vi "Final_Write_Key.vi"(7 "AllObjs[]":refnum<vi>[](array[refnum]), 8 "error in (no error)":errorcluster, 9 "Label.Text":string, 10 "String":string, 11 "Refnum in":T1) -> (0 "error out":errorcluster, 3 "Refnum out":T1)   [LabVIEW 2014]
uses:
  <vilib>/Utility/config.llb/Config Data RefNum.ctl
  <vilib>/Utility/config.llb/Write Key (Double).vi
  <vilib>/Utility/config.llb/Write Key (String).vi
  <vilib>/Utility/config.llb/Write Key (Path).vi
  <vilib>/Utility/config.llb/Write Key (I32).vi
  <vilib>/Utility/config.llb/Write Key (U32).vi
  <vilib>/Utility/config.llb/Write Key (Boolean).vi
  <vilib>/Utility/config.llb/NI_LVConfig.lvlib
  <vilib>/Utility/VariantDataType/VariantType.lvlib
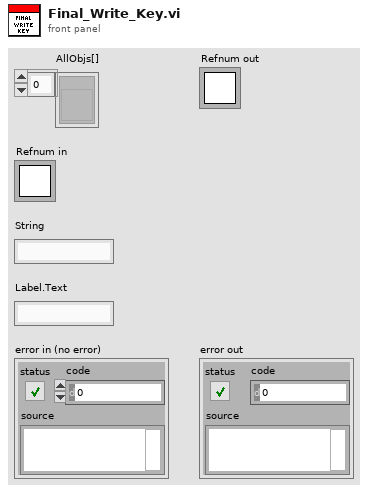
[diagram p1: front panel]
types:
  T1 = typedef "NI_LVConfig.lvlib/Config Data RefNum.ctl" = refnum<k1>
  T2 = typedef "VariantType.lvlib/Type.ctl" = enum8{"Invalid Type", "Void", "I8", "I16", "I32", "I64", "U8", "U16", "U32", "U64", "Single Float", "Double Float", "Extended Float", "Single Complex", "Double Complex", "Extended Complex", "Enum U8", "Enum U16", "Enum U32", "Enum U64", "Single Float With Unit", "Double Float With Unit", "Extended Float With Unit", "Single Complex with Unit", "Double Complex with Unit", "Extended Complex with Unit", "Boolean", "String", "Path", "Picture", "Tag", "Array", "Cluster", "Variant", "LV Variant", "Waveform", "Timestamp", "Digital Waveform", "Digital Data", "ExpressData", "Refnum", "External Data", "VI", "Poly VI", "LabVIEW Class Instance", "Fixed Point"}
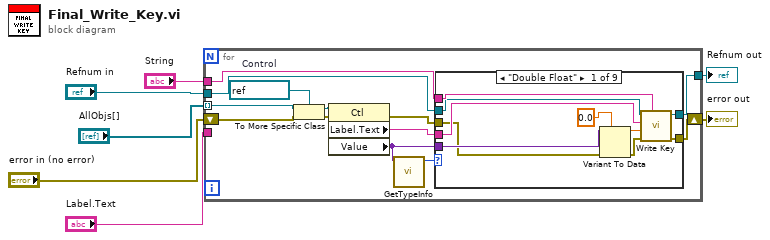
[diagram p0: block diagram]
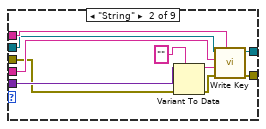
[diagram p2: hidden frame]
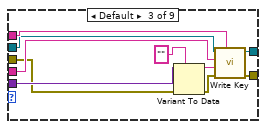
[diagram p3: hidden frame]
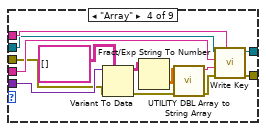
[diagram p4: hidden frame]
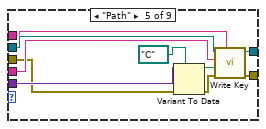
[diagram p5: hidden frame]
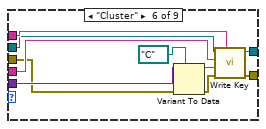
[diagram p6: hidden frame]
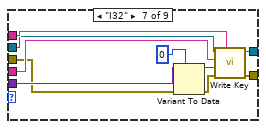
[diagram p7: hidden frame]
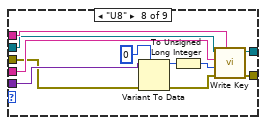
[diagram p8: hidden frame]
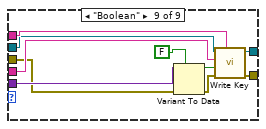
[diagram p9: hidden frame]
diagram:
  n1 = for {
    tunnel: "String" -> [w20]
    tunnel: [w19] -> w1
    tunnel: "Refnum in" -> [w15]
    tunnel: "AllObjs[]" -> [w11] mode=indexing
    tunnel: "Label.Text" -> [_]
    shift-right: [w18] -> w2
    shift-left: "error in (no error)" -> [w10]
    w17 = refnum<vi> refnum  # Control
    n2 = To More Specific Class(target class=w17, reference=w11, error in=w10) -> (specific class reference=w16:refnum<vi>, error out=w9:errorcluster)
    n3 = property class="Ctl"(reference=w16, error in=w9) -> (error out=w8:errorcluster, "Label.Text"=w12:string, "Value"=w13:variant)  [unwired: 1 out]
    n4 = call <vilib>:"GetTypeInfo.vi"("Variant"=w13) -> ("Type Enum"=w14:T2)  [unwired: 6 in, 4 out]
    n5 = case shown="\"Double Float\"" w14 {
      tunnel: w20 -> [w30 w40 w50 w63 w67 w83 w93 w104 w114]
      tunnel: w12 -> [w29 w39 w43 w62 w66 w82 w92 w103 w113]
      tunnel: w13 -> [w28 w38 w49 w61 w73 w81 w91 w102 w112]
      tunnel: w15 -> [w23 w33 w44 w56 w68 w76 w85 w96 w107]
      tunnel: [w27 w37 w48 w60 w72 w80 w90 w101 w111] -> w18
      tunnel: [w26 w36 w47 w59 w71 w79 w89 w100 w110] -> w19
      tunnel: w8 -> [w22 w32 w42 w53 w65 w75 w84 w95 w106]
      frame "Double Float" {
        n6 = Variant To Data(error in=w22, type=0.0, Variant=w28) -> (data=w24:dbl, error out=w21:errorcluster)
        n7 = call-poly <vilib>:"Write Key.vi"("section"=w30, "error in (no error)"=w21, "value"=w24, "key"=w29, "refnum"=w23) -> ("error out"=w27:errorcluster, "refnum out"=w26:T1)  [unwired: 4 in, 1 out]
      }
      frame "String" {
        n8 = Variant To Data(error in=w32, type="" ("Label.Text"), Variant=w38) -> (data=w34:string, error out=w31:errorcluster)
        n9 = call-poly <vilib>:"Write Key.vi"("section"=w40, "error in (no error)"=w31, "value"=w34, "key"=w39, "refnum"=w33) -> ("error out"=w37:errorcluster, "refnum out"=w36:T1)  [unwired: 4 in, 1 out]
      }
      frame Default {
        n10 = Variant To Data(error in=w42, type="" ("Label.Text"), Variant=w49) -> (data=w45:string, error out=w41:errorcluster)
        n11 = call-poly <vilib>:"Write Key.vi"("section"=w50, "error in (no error)"=w41, "value"=w45, "key"=w43, "refnum"=w44) -> ("error out"=w48:errorcluster, "refnum out"=w47:T1)  [unwired: 4 in, 1 out]
      }
      frame "Array" {
        n12 = Variant To Data(error in=w53, type=string[][] [], Variant=w61) -> (data=w57:string[][], error out=w52:errorcluster)
        n13 = Fract/Exp String To Number(string=w57) -> (number=w55:dbl[][])  [unwired: 3 in, 1 out]
        n14 = call "UTILITY DBL Array to String Array.vi"("Error in (no error)"=w52, "Array in"=w55) -> ("Error out"=w51:errorcluster, "String array out"=w54:string)  [unwired: 8 in]
        n15 = call-poly <vilib>:"Write Key.vi"("section"=w63, "error in (no error)"=w51, "value"=w54, "key"=w62, "refnum"=w56) -> ("error out"=w60:errorcluster, "refnum out"=w59:T1)  [unwired: 4 in, 1 out]
      }
      frame "Path" {
        n16 = Variant To Data(error in=w65, type=path "C:/" ("configuration file path 2"), Variant=w73) -> (data=w69:path, error out=w64:errorcluster)
        n17 = call-poly <vilib>:"Write Key.vi"("section"=w67, "error in (no error)"=w64, "value"=w69, "key"=w66, "refnum"=w68) -> ("error out"=w72:errorcluster, "refnum out"=w71:T1)  [unwired: 4 in, 1 out]
      }
      frame "Cluster" {
        n18 = Variant To Data(error in=w75, type=path "C:/" ("configuration file path 2"), Variant=w81) -> (data=w77:path, error out=w74:errorcluster)
        n19 = call-poly <vilib>:"Write Key.vi"("section"=w83, "error in (no error)"=w74, "value"=w77, "key"=w82, "refnum"=w76) -> ("error out"=w80:errorcluster, "refnum out"=w79:T1)  [unwired: 4 in, 1 out]
      }
      frame "I32" {
        n20 = Variant To Data(error in=w84, type=0, Variant=w91) -> (data=w86:i32, error out=w87:errorcluster)
        n21 = call-poly <vilib>:"Write Key.vi"("section"=w93, "error in (no error)"=w87, "value"=w86, "key"=w92, "refnum"=w85) -> ("error out"=w90:errorcluster, "refnum out"=w89:T1)  [unwired: 4 in, 1 out]
      }
      frame "U8" {
        n22 = Variant To Data(error in=w95, type=u8 0, Variant=w102) -> (data=w99:u8, error out=w94:errorcluster)
        n23 = To Unsigned Long Integer(number=w99) -> (unsigned 32bit integer=w97:u32)
        n24 = call-poly <vilib>:"Write Key.vi"("section"=w104, "error in (no error)"=w94, "value"=w97, "key"=w103, "refnum"=w96) -> ("error out"=w101:errorcluster, "refnum out"=w100:T1)  [unwired: 4 in, 1 out]
      }
      frame "Boolean" {
        n25 = Variant To Data(error in=w106, type=FALSE ("Write? 2"), Variant=w112) -> (data=w109:bool, error out=w105:errorcluster)
        n26 = call-poly <vilib>:"Write Key.vi"("section"=w114, "error in (no error)"=w105, "value"=w109, "key"=w113, "refnum"=w107) -> ("error out"=w111:errorcluster, "refnum out"=w110:T1)  [unwired: 4 in, 1 out]
      }
    }
  }
  "error out" <- w2
  "Refnum out" <- w1
